vi "Do.vi"(8 "error in (no error)":errorcluster, 10 "Actor in":refnum<class "Actor.lvclass">, 11 "Main UI Task Msg":refnum<class "Main UI Task Msg.lvclass">) -> (0 "error out":errorcluster, 2 "Actor out":refnum<class "Actor.lvclass">)   [LabVIEW 2016, in "Main UI Actor.lvlib" / "Main UI Task Msg.lvclass"]
uses:
  Main UI Task Msg.lvclass
  <vilib>/ActorFramework/Actor/Actor.lvclass
  Main UI/Main UI.lvclass
  E:/Program Files (x86)/National Instruments/LabVIEW 2016/vi.lib/ActorFramework/Actor/Actor.lvclass
  Main UI Task Msg.lvclass/Main UI Task Msg.ctl
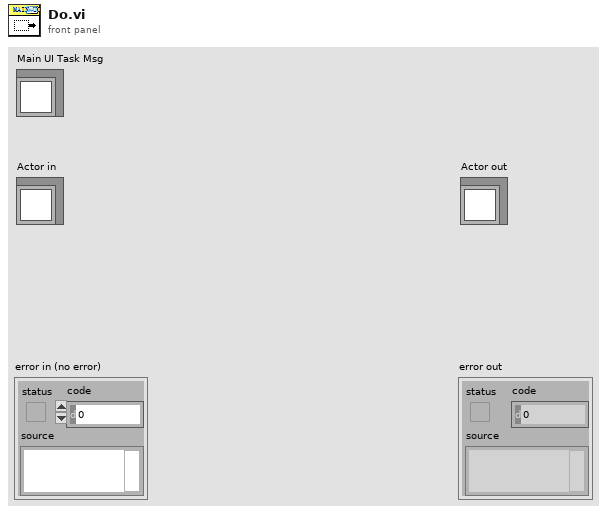
[diagram p1: front panel]
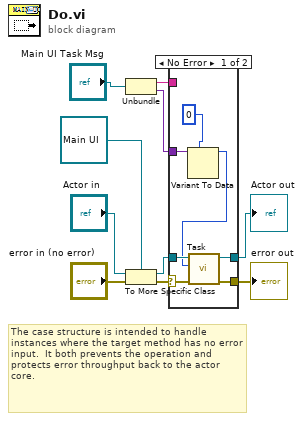
[diagram p0: block diagram]
diagram:
  # "The case structure is intended to handle instances where the target method has no error input.  It both prevents the operation and protects error throughput back to the actor core."
  n1 = Unbundle("Main UI Task Msg") -> (w2:string, w1:variant)
  n2 = To More Specific Class(target class=refnum<class "Main UI.lvclass"> refnum ("Actor in"), reference="Actor in", error in="error in (no error)") -> (specific class reference=w9:refnum<class "Main UI.lvclass">, error out=w5:errorcluster)
  n3 = case shown="No Error" w5 {
    selector: w5 -> [w14 w19]
    tunnel: w9 -> [w17 w18]
    tunnel: [w16 w19] -> w4
    tunnel: [w15 w18] -> w3
    tunnel: w2 -> [_ _]
    tunnel: w1 -> [w13 _]
    frame No Error {
      n4 = Variant To Data(type=0, Variant=w13) -> (data=w11:i32)  [unwired: 1 in, 1 out]
      n5 = call-dynamic "Task.vi"("error in (no error)"=w14, "Data"=w11, "Main UI in"=w17) -> ("error out"=w16:errorcluster, "Main UI out"=w15:refnum<class "Main UI.lvclass">)  [unwired: 7 in]
    }
    frame Error {
    }
  }
  "error out" <- w4
  "Actor out" <- w3
